vi "Setup.vi"(10 "Setup":refnum<class "Setup.lvclass">, 11 "Core Actor in":refnum<class "Core Actor.lvclass">) -> (0 "Error out":errorcluster, 3 "Core Actor out":refnum<class "Core Actor.lvclass">)   [LabVIEW 2025, in "jettl.lvlib" / "Core Actor.lvlib" / "Core Actor.lvclass"]
uses:
  Core Actor.lvclass
  Setup/Setup/Setup.lvclass
  Attributes.ctl
  Transport/Transport/Transport.lvclass
  Attributes/Attributes/Attributes.lvclass
  Refs/Refs.lvclass
  Msg Set.ctl
  Msg/Msg.lvclass
  Actor/Actor.lvclass
  Core Actor.lvclass/Core Actor.ctl
  Attributes/Attributes.lvlib
  jettl.lvlib
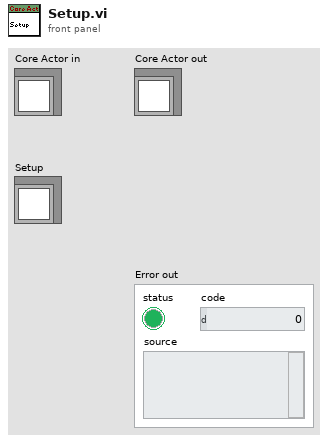
[diagram p1: front panel]
types:
  T1 = typedef "jettl.lvlib/Attributes.ctl" = cluster{"UID":string, "Transport":refnum<class "Transport.lvclass">, "Unified Msg Set":T2, "Actor Ref":refnum<vi>, "Application Ref":refnum<vi>, "Parent Attributes":refnum<class "Attributes.lvclass">, "Root":bool, "Persistent Layers":refnum<class "Actor.lvclass">[], "Refs":refnum<class "Refs.lvclass">}
  T2 = typedef "jettl.lvlib/Msg Set.ctl" = set{refnum<class "Msg.lvclass">}
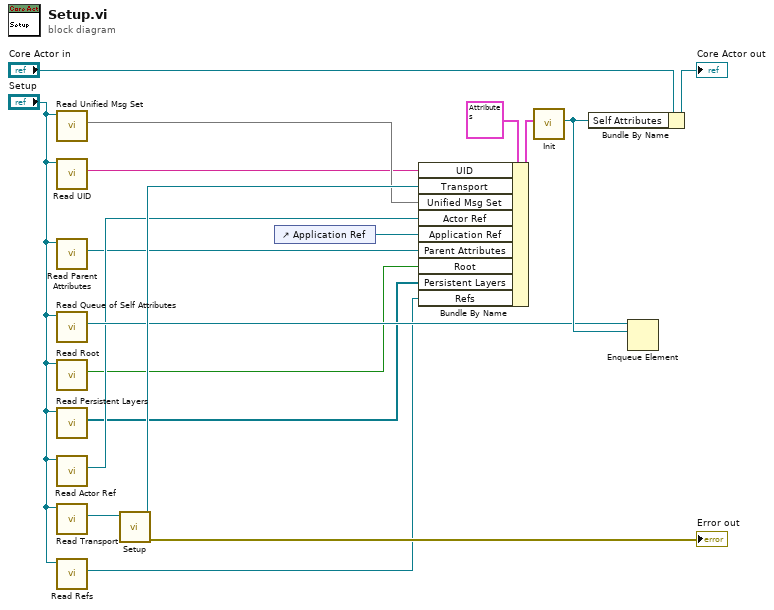
[diagram p0: block diagram]
diagram:
  n1 = call-dynamic "Read Unified Msg Set.vi"("Setup in"="Setup") -> ("Unified Msg Set"=w10:T2)  [unwired: 10 in]
  n2 = call-dynamic "Read UID.vi"("Setup in"="Setup") -> ("UID"=w7:string)  [unwired: 10 in]
  n3 = call-dynamic "Read Parent Attributes.vi"("Setup in"="Setup") -> ("Parent Attributes"=w5:refnum<class "Attributes.lvclass">)  [unwired: 10 in]
  n4 = call-dynamic "Read Queue of Self Attributes.vi"("Setup in"="Setup") -> ("Queue of Self Attributes"=w9:refnum<queue>)  [unwired: 10 in]
  n5 = call-dynamic "Read Root.vi"("Setup in"="Setup") -> ("Root"=w4:bool)  [unwired: 10 in]
  n6 = call-dynamic "Read Persistent Layers.vi"("Setup in"="Setup") -> ("Persistent Layers"=w3:refnum<class "Actor.lvclass">[])  [unwired: 10 in]
  n7 = call-dynamic "Read Actor Ref.vi"("Setup in"="Setup") -> ("Actor Ref"=w8:refnum<vi>)  [unwired: 10 in]
  n8 = call-dynamic "Read Transport.vi"("Setup in"="Setup") -> ("Transport"=w6:refnum<class "Transport.lvclass">)  [unwired: 10 in]
  n9 = call-dynamic "Read Refs.vi"("Setup in"="Setup") -> ("Refs"=w1:refnum<class "Refs.lvclass">)  [unwired: 10 in]
  n10 = call-dynamic "Setup.vi"("Transport in"=w6) -> ("Error out"=→"Error out":errorcluster, "Transport out"=w11:refnum<class "Transport.lvclass">)  [unwired: 9 in]
  n11 = control-ref of="Application Ref"() -> (w14:refnum<vi>)
  n12 = Bundle By Name(cluster=T1 {"UID"="", "Transport"=refnum, "Unified Msg Set"={}, "Actor Ref"=refnum, "Application Ref"=refnum, "Parent Attributes"=refnum, "Root"=FALSE, "Persistent Layers"=[], "Refs"=refnum} ("Attributes"), "UID"=w7, "Transport"=w11, "Unified Msg Set"=w10, "Actor Ref"=w8, "Application Ref"=w14, "Parent Attributes"=w5, "Root"=w4, "Persistent Layers"=w3, "Refs"=w1) -> (w13:T1)
  n13 = call "Init.vi"("Attributes"=w13) -> ("Attributes"=w16:refnum<class "Attributes.lvclass">)  [unwired: 10 in]
  n14 = Bundle By Name(cluster="Core Actor in", "Self Attributes"=w16) -> (→"Core Actor out":refnum<class "Core Actor.lvclass">)
  n15 = Enqueue Element(queue=w9, element=w16) -> ()  [unwired: 2 in, 3 out]
